vi "Trust Unknown Server Identity.vi"(8 "error in (no error)":errorcluster, 11 "client in":refnum<class "Generic Client.lvclass">) -> (0 "error out":errorcluster, 2 "permanent?":bool, 3 "client out":refnum<class "Generic Client.lvclass">)   [LabVIEW 2020, in "NI_SSH.lvlib" / "Generic Client.lvclass"]
doc: "Explicitly trust the identity of a server that is currently unknown.\n\nThis can only be called after an SFTP connection attempt has failed. Otherwise, this VI will return an error."
uses:
  <vilib>/net/SSH/Client/Generic/Generic Client.lvclass
  <vilib>/net/SSH/Client/Generic/Generic Client.lvclass/Generic Client.ctl
  <vilib>/net/SSH/Client/Generic/Read untrusted fingerprint is incorrect_.vi
  <vilib>/Utility/error.llb/Error Cluster From Error Code.vi
  <vilib>/ErrorRing/Error Ring.xnode
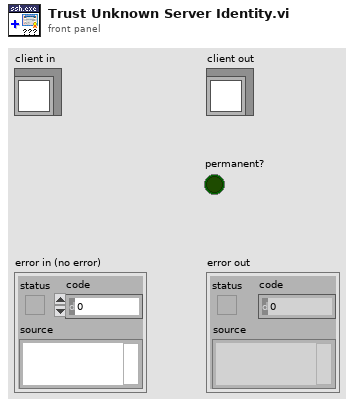
[diagram p1: front panel]
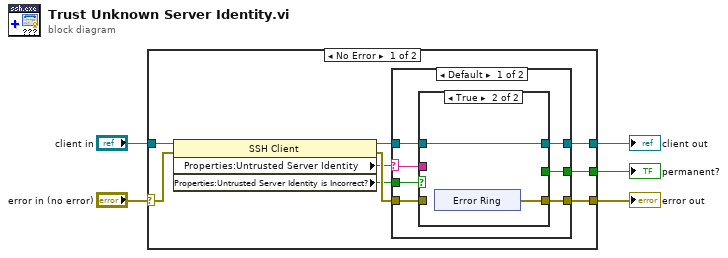
[diagram p0: block diagram]
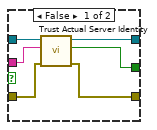
[diagram p2: hidden frame]
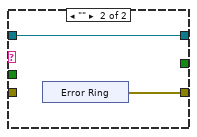
[diagram p3: hidden frame]
diagram:
  n1 = case shown="No Error" "error in (no error)" {
    selector: "error in (no error)" -> [w10 w41]
    tunnel: [w13 w41] -> w1
    tunnel: "client in" -> [w11 w40]
    tunnel: [w14 w40] -> w3
    tunnel: [w6 _] -> w4
    frame No Error {
      n2 = property class="SSH Client"(reference=w11, error in=w10) -> (reference out=w12:refnum<class "Generic Client.lvclass">, error out=w9:errorcluster, "Properties:Untrusted Server Identity"=w8:string, "Properties:Untrusted Server Identity is Incorrect?"=w7:bool)
      n3 = case shown="Default" w8 {
        selector: w8 -> [w20 _]
        tunnel: w12 -> [w21 w35]
        tunnel: [w19 w35] -> w14
        tunnel: w9 -> [w16 _]
        tunnel: [w17 w34] -> w13
        tunnel: w7 -> [w18 _]
        tunnel: [w15 _] -> w6
        frame Default {
          n4 = case shown="True" w18 {
            tunnel: w21 -> [w27 w29]
            tunnel: w20 -> [w26 _]
            tunnel: [w23 w29] -> w19
            tunnel: [w24 w28] -> w17
            tunnel: w16 -> [w25 _]
            tunnel: [w22 _] -> w15
            frame False {
              n5 = call-dynamic "Trust Actual Server Identity.vi"("error in (no error)"=w25, "fingerprint"=w26, "SSH Client in"=w27) -> ("error out"=w24:errorcluster, "permanent?"=w22:bool, "SSH Client out"=w23:refnum<class "Generic Client.lvclass">)  [unwired: 6 in]
            }
            frame True {
              n6 = xnode "Error Ring"() -> ("error out"=w28:errorcluster)
            }
          }
        }
        frame "" {
          n7 = xnode "Error Ring"() -> ("error out"=w34:errorcluster)
        }
      }
    }
    frame Error {
    }
  }
  "error out" <- w1
  "client out" <- w3
  "permanent?" <- w4
